vi "Device tester (juicer).vi"() -> ()   [LabVIEW 2015]
uses:
  Device/Typedefs/Juicer.ctl
  Rack/Typedefs/OutputRequest refnum.ctl
  Rack/Typedefs/OutputRequest.ctl
  Rack/Typedefs/InputData cluster.ctl
  Rack/Methods/Port drivers/DigitalInput-DataCluster.ctl
  Device/Typedefs/Valve.ctl
  Rack/Methods/Rack-Init.vi
  Device/Methods/Juicer-Init.vi
  Device/Methods/Valve-Init.vi
  Rack/Methods/Rack-Config.vi
  Rack/Methods/Rack-Start.vi
  Device/Methods/Valve-Open.vi
  Device/Methods/Valve-Close.vi
  Device/Methods/Valve-Pulse.vi
  Device/Methods/Juicer-ChangeMode.vi
  Rack/Methods/Rack-Stop.vi
panel:
  in  "Valve #":i32=1
  out "Valve refs":refnum<vi>[](array[refnum])
  in  "Valve 12":T1={"Settings"={"Timestamp port name"="dsub_panel.p9.7", "Port name"="juicer.valve12", "Port index"=-1}, "OutputRequest event ref"=refnum, "InputData reference"=refnum, "Default length (ms)"=100}
  in  "Valve 11":T1={"Settings"={"Timestamp port name"="dsub_panel.p9.7", "Port name"="juicer.valve11", "Port index"=-1}, "OutputRequest event ref"=refnum, "InputData reference"=refnum, "Default length (ms)"=100}
  in  "Valve 10":T1={"Settings"={"Timestamp port name"="dsub_panel.p9.7", "Port name"="juicer.valve10", "Port index"=-1}, "OutputRequest event ref"=refnum, "InputData reference"=refnum, "Default length (ms)"=100}
  in  "Valve 9":T1={"Settings"={"Timestamp port name"="dsub_panel.p9.7", "Port name"="juicer.valve9", "Port index"=-1}, "OutputRequest event ref"=refnum, "InputData reference"=refnum, "Default length (ms)"=100}
  in  "Valve 8":T1={"Settings"={"Timestamp port name"="dsub_panel.p9.7", "Port name"="juicer.valve8", "Port index"=-1}, "OutputRequest event ref"=refnum, "InputData reference"=refnum, "Default length (ms)"=100}
  in  "Valve 7":T1={"Settings"={"Timestamp port name"="dsub_panel.p9.7", "Port name"="juicer.valve7", "Port index"=-1}, "OutputRequest event ref"=refnum, "InputData reference"=refnum, "Default length (ms)"=100}
  in  "Valve 6":T1={"Settings"={"Timestamp port name"="dsub_panel.p9.7", "Port name"="juicer.valve6", "Port index"=-1}, "OutputRequest event ref"=refnum, "InputData reference"=refnum, "Default length (ms)"=100}
  in  "Valve 5":T1={"Settings"={"Timestamp port name"="dsub_panel.p9.7", "Port name"="juicer.valve5", "Port index"=-1}, "OutputRequest event ref"=refnum, "InputData reference"=refnum, "Default length (ms)"=100}
  in  "Valve 4":T1={"Settings"={"Timestamp port name"="dsub_panel.p9.7", "Port name"="juicer.valve4", "Port index"=-1}, "OutputRequest event ref"=refnum, "InputData reference"=refnum, "Default length (ms)"=100}
  in  "Valve 3":T1={"Settings"={"Timestamp port name"="dsub_panel.p9.7", "Port name"="juicer.valve3", "Port index"=-1}, "OutputRequest event ref"=refnum, "InputData reference"=refnum, "Default length (ms)"=100}
  in  "Valve 2":T1={"Settings"={"Timestamp port name"="dsub_panel.p9.7", "Port name"="juicer.valve2", "Port index"=-1}, "OutputRequest event ref"=refnum, "InputData reference"=refnum, "Default length (ms)"=100}
  in  "Valve 1":T1={"Settings"={"Timestamp port name"="BNC_panel.P0.0", "Port name"="BNC_panel.P0.1", "Port index"=-1}, "OutputRequest event ref"=refnum, "InputData reference"=refnum, "Default length (ms)"=100}
  in  "Juicer":T3={"Mode"=enum."Off", "Settings"={"Bleed #1 port index"=-1, "Bleed #1 port name"="juicer.bleed1", "Bleed #2 port name"="juicer.bleed2", "Bleed #2 port index"=-1, "Flush port name"="juicer.flush", "Flush port index"=-1, "Purge port name"="juicer.purge", "Purge port index"=-1, "Timestamp port name"="dsub_panel.p9.7"}, "OutputRequest event ref"=refnum, "InputData reference"=refnum}
  in  "# repeats":u32=200
  in  "Serial pulse":bool
  in  "Juicer mode":enum16{"off", "reward", "flush", "purge"}(ring)
  in  "Duration (0 for default)":i32
  in  "stop":bool
  in  "Close all":bool
  in  "Close":bool
  in  "Open":bool
  in  "Pulse":bool
  # "Remember to stop this VI before starting\nother behavior VIs that use the juicer!"
  # "(must be on same NI card)"
  # "(must be on same NI card)"
  # "(must be on same NI card)"
  # "(must be on same NI card)"
  # "(must be on same NI card)"
  # "(must be on same NI card)"
  # "(must be on same NI card)"
  # "(must be on same NI card)"
  # "(must be on same NI card)"
  # "(must be on same NI card)"
  # "(must be on same NI card)"
  # "(must be on same NI card)"
  # "(must be on same NI card)"
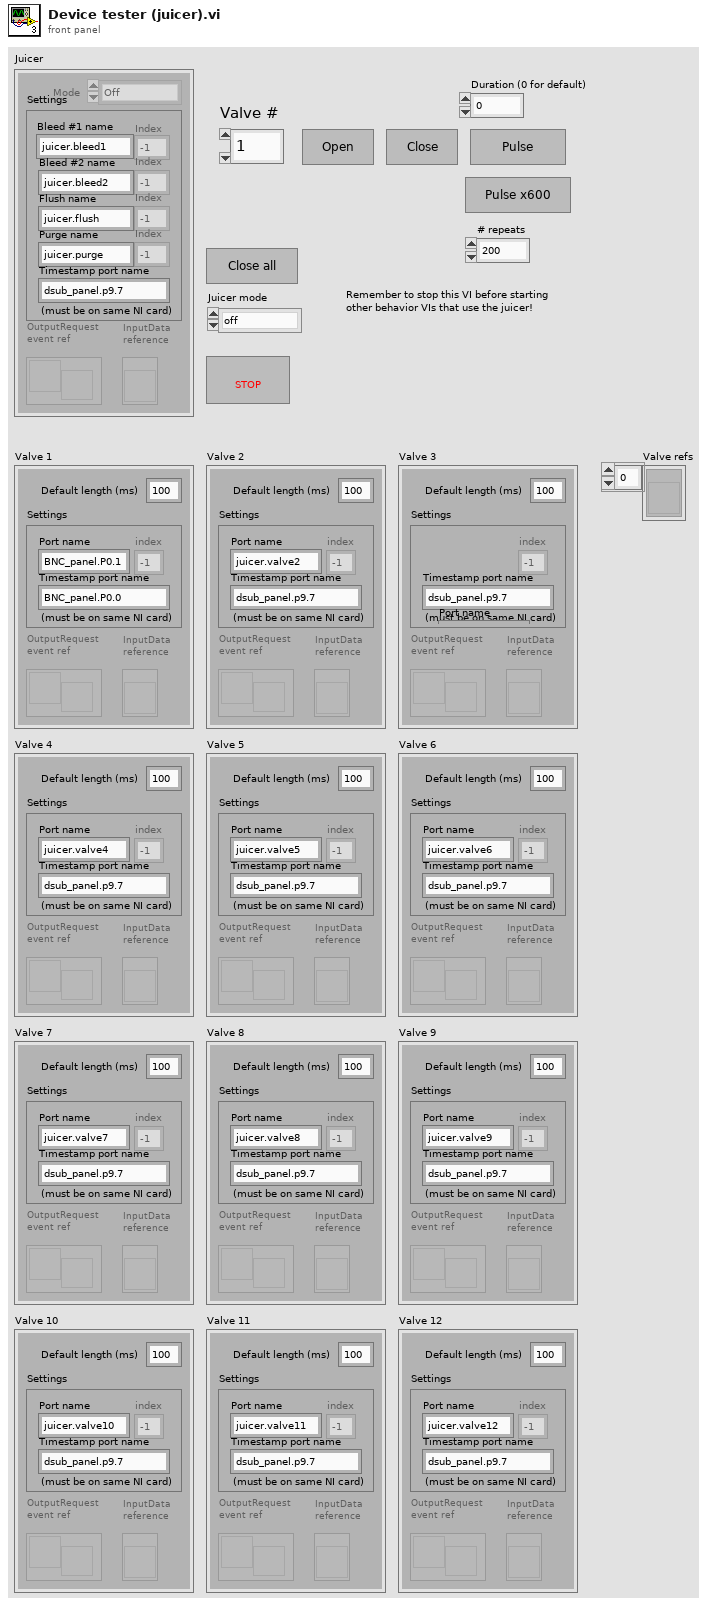
[diagram p1: front panel]
types:
  T1 = typedef "Valve.ctl" = cluster{"Settings":cluster{"Timestamp port name":string, "Port name":string, "Port index":i32}, "OutputRequest event ref":T2, "InputData reference":refnum<vi>, "Default length (ms)":i32}
  T2 = typedef "OutputRequest refnum.ctl" = refnum<user-event>
  T3 = typedef "Juicer.ctl" = cluster{"Mode":enum16{"Off", "Juice/reward", "Water flush", "Air purge"}, "Settings":cluster{"Bleed #1 port index":i32, "Bleed #1 port name":string, "Bleed #2 port name":string, "Bleed #2 port index":i32, "Flush port name":string, "Flush port index":i32, "Purge port name":string, "Purge port index":i32, "Timestamp port name":string}, "OutputRequest event ref":T2, "InputData reference":refnum<vi>}
  T4 = typedef "Rack driver configuration cluster.ctl" = cluster{"DigitalInput":T5, "DigitalOutput":T6, "FileOutput":T7, "AnalogOutput":T8, "DataSocketOutput":T9}
  T5 = typedef "DigitalInput-Configuration.ctl" = cluster{"Lines":tag[], "Refresh period (ms)":u32}
  T6 = typedef "DigitalOutput-Configuration.ctl" = cluster{"Output Lines":tag[], "DO timestamp lines":tag[], "Timestamp lines":tag[]}
  T7 = typedef "FileOutput-Configuration.ctl" = cluster{"Logfile path":path}
  T8 = typedef "AnalogOutput-Configuration.ctl" = cluster{"Output Lines":tag[], "AO timestamp lines":tag[]}
  T9 = typedef "DataSocketOutput-Configuration.ctl" = cluster{"DataSocket URL":string}
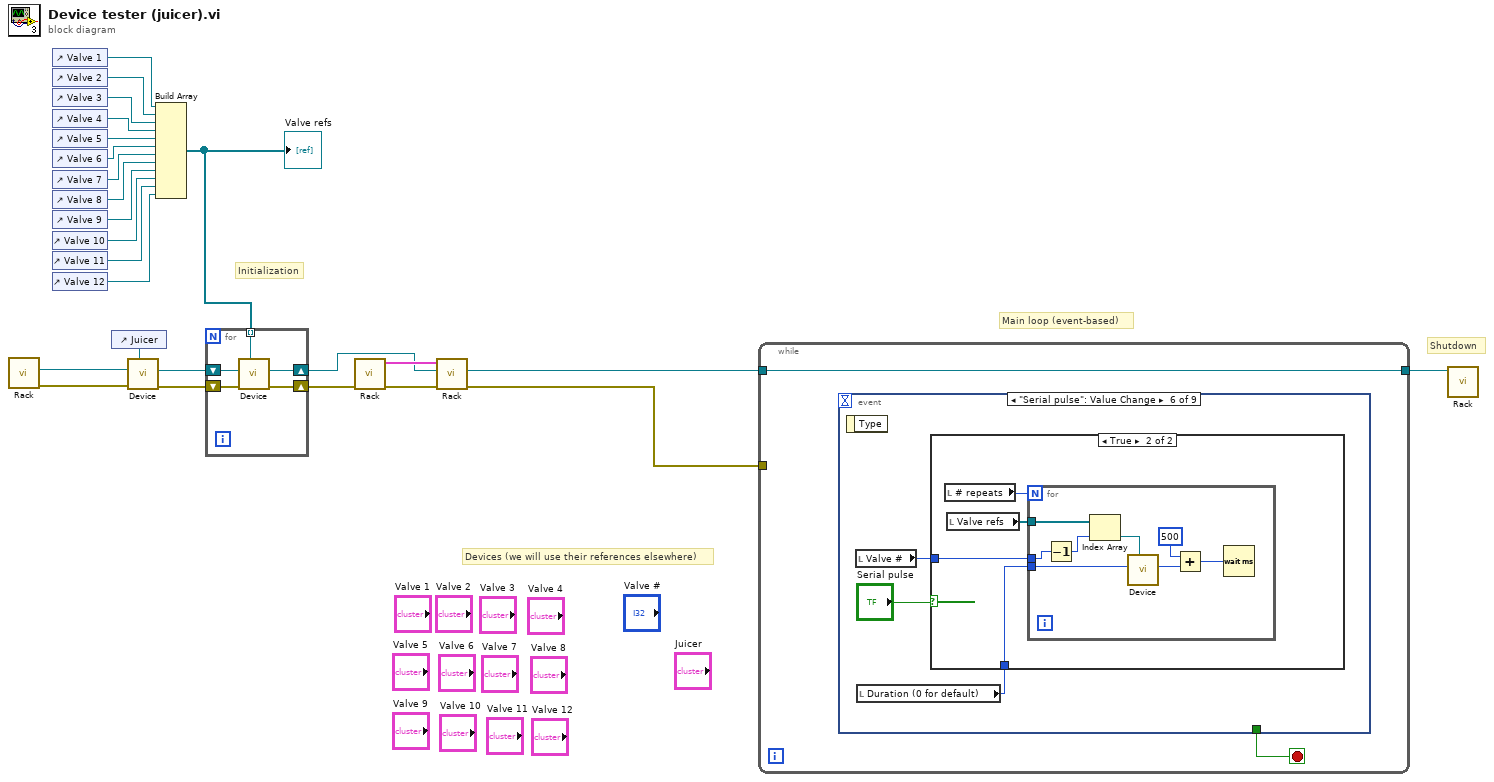
[diagram p0: block diagram]
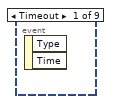
[diagram p2: hidden frame]
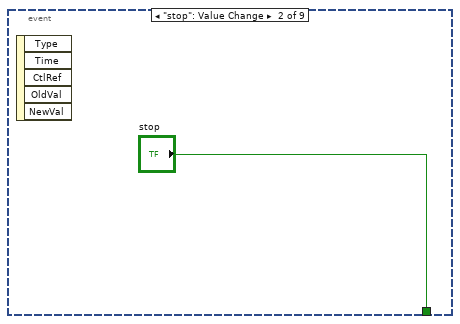
[diagram p3: hidden frame]
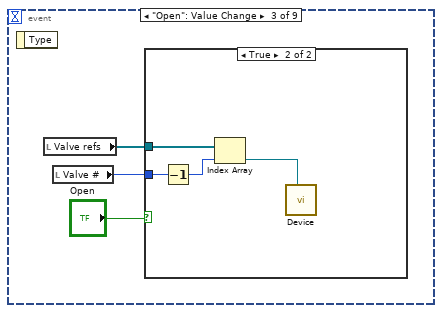
[diagram p4: hidden frame]
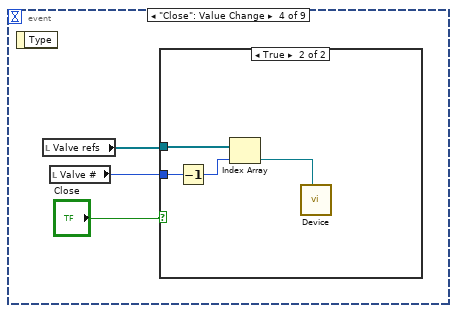
[diagram p6: hidden frame]
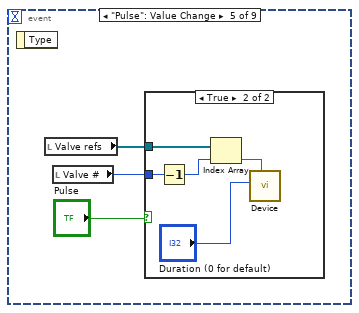
[diagram p8: hidden frame]
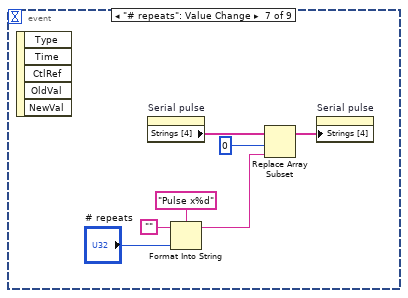
[diagram p11: hidden frame]
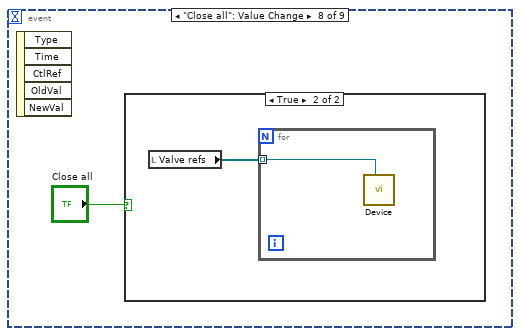
[diagram p12: hidden frame]
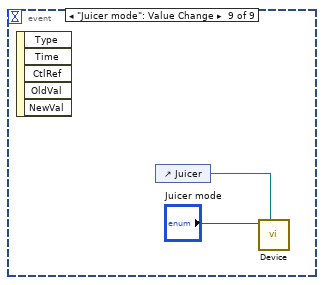
[diagram p14: hidden frame]
diagram:
  # "Main loop (event-based)"
  # "Shutdown"
  # "Initialization"
  # "Devices (we will use their references elsewhere)"
  n1 = call-poly "Rack.vi"() -> ("error out"=w25:errorcluster, "OutputRequest\nevent ref"=w21:T2)  [unwired: 10 in]
  n2 = control-ref of="Valve 1"() -> (w18:refnum<vi>)
  n3 = control-ref of="Valve 2"() -> (w17:refnum<vi>)
  n4 = control-ref of="Valve 3"() -> (w16:refnum<vi>)
  n5 = control-ref of="Valve 4"() -> (w15:refnum<vi>)
  n6 = control-ref of="Valve 5"() -> (w14:refnum<vi>)
  n7 = control-ref of="Valve 6"() -> (w7:refnum<vi>)
  n8 = control-ref of="Valve 7"() -> (w8:refnum<vi>)
  n9 = control-ref of="Valve 8"() -> (w9:refnum<vi>)
  n10 = control-ref of="Valve 9"() -> (w10:refnum<vi>)
  n11 = control-ref of="Valve 10"() -> (w11:refnum<vi>)
  n12 = control-ref of="Valve 11"() -> (w12:refnum<vi>)
  n13 = control-ref of="Valve 12"() -> (w13:refnum<vi>)
  n14 = control-ref of="Juicer"() -> (w19:refnum<vi>)
  n15 = call-poly "Device.vi"("Device reference"=w19, "error in (no error)"=w25, "OutputRequest event ref"=w21) -> ("error out"=w6:errorcluster, "OutputRequest (dup)"=w4:T2)  [unwired: 6 in, 1 out]
  n16 = Build Array(w18, w17, w16, w15, w14, w7, w8, w9, w10, w11, w12, w13) -> (w1:refnum<vi>[])
  "Valve refs" <- w1
  n17 = for {
    shift-right: [w27] -> w5
    shift-left: w6 -> [w30]
    shift-right: [w28] -> w3
    shift-left: w4 -> [w29]
    tunnel: w1 -> [w26] mode=indexing
    n18 = call-poly "Device.vi"("Device reference"=w26, "error in (no error)"=w30, "OutputRequest event ref"=w29) -> ("error out"=w27:errorcluster, "OutputRequest (dup)"=w28:T2)  [unwired: 6 in, 1 out]
  }
  n19 = call-poly "Rack.vi"("error in (no error)"=w5) -> ("error out"=w24:errorcluster, "Configuration"=w23:T4)  [unwired: 9 in]
  n20 = call-poly "Rack.vi"("error in (no error)"=w24, "OutputRequest event ref"=w3, "Configuration"=w23) -> ("error out"=w2:errorcluster, "OutputRequest event ref (dup)"=w20:T2)  [unwired: 7 in]
  n21 = while {
    tunnel: w20 -> [w31]
    tunnel: [w31] -> w22
    tunnel: w2 -> [_]
    stop <- w32 stop-if-true
    n22 = event shown="[5] \"Serial pulse\": Value Change" {
      selector: _ -> [_ _ _ _ _ _ _ _ _]
      dyn-events: _ -> [_ _ _ _ _ _ _ _ _]
      timeout: _ -> [_ _ _ _ _ _ _ _ _]
      tunnel: [_ "stop" _ _ _ _ _ _ _] -> w32
      event Timeout {
        n23 = event-data() -> ()  [unwired: 1 in, 2 out]
      }
      event "stop": Value Change {
        n24 = event-data() -> ()  [unwired: 1 in, 5 out]
      }
      event "Open": Value Change {
        n25 = event-data() -> ()  [unwired: 1 in, 1 out]
        n26 = local read "Valve refs"() -> (w34:refnum<vi>[])
        n27 = local read "Valve #"() -> (w35:i32)
        n28 = case shown="True" "Open" {
          tunnel: w35 -> [_ w39]
          tunnel: w34 -> [_ w40]
          frame False {
          }
          frame True {
            n29 = Decrement(x=w39) -> (x-1=w38:i32)
            n30 = Index Array(array=w40, index=w38) -> (element=w37:refnum<vi>)
            n31 = call-poly "Device.vi"("Device reference"=w37) -> ()  [unwired: 10 in, 1 out]
          }
        }
      }
      event "Close": Value Change {
        n32 = event-data() -> ()  [unwired: 1 in, 1 out]
        n33 = local read "Valve refs"() -> (w41:refnum<vi>[])
        n34 = local read "Valve #"() -> (w42:i32)
        n35 = case shown="True" "Close" {
          tunnel: w42 -> [_ w46]
          tunnel: w41 -> [_ w47]
          frame False {
          }
          frame True {
            n36 = Decrement(x=w46) -> (x-1=w45:i32)
            n37 = Index Array(array=w47, index=w45) -> (element=w44:refnum<vi>)
            n38 = call-poly "Device.vi"("Device reference"=w44) -> ()  [unwired: 10 in, 1 out]
          }
        }
      }
      event "Pulse": Value Change {
        n39 = event-data() -> ()  [unwired: 1 in, 1 out]
        n40 = local read "Valve refs"() -> (w48:refnum<vi>[])
        n41 = local read "Valve #"() -> (w50:i32)
        n42 = case shown="True" "Pulse" {
          tunnel: w50 -> [_ w53]
          tunnel: w48 -> [_ w51]
          frame False {
          }
          frame True {
            n43 = Decrement(x=w53) -> (x-1=w54:i32)
            n44 = Index Array(array=w51, index=w54) -> (element=w52:refnum<vi>)
            n45 = call-poly "Device.vi"("Device reference"=w52, "Duration"="Duration (0 for default)") -> ()  [unwired: 8 in, 2 out]
          }
        }
      }
      event "Serial pulse": Value Change {
        n46 = event-data() -> ()  [unwired: 1 in, 1 out]
        n47 = local read "Valve #"() -> (w58:i32)
        n48 = local read "Duration (0 for default)"() -> (w56:i32)
        n49 = case shown="True" "Serial pulse" {
          tunnel: w58 -> [_ w62]
          tunnel: w56 -> [_ w61]
          frame False {
          }
          frame True {
            n50 = local read "# repeats"() -> (w60:u32)
            n51 = local read "Valve refs"() -> (w59:refnum<vi>[])
            n52 = for {
              N: w60 -> [_]
              tunnel: w62 -> [w65]
              tunnel: w61 -> [w70]
              tunnel: w59 -> [w64]
              n53 = Decrement(x=w65) -> (x-1=w66:i32)
              n54 = Index Array(array=w64, index=w66) -> (element=w63:refnum<vi>)
              n55 = call-poly "Device.vi"("Device reference"=w63, "Duration"=w70) -> ("Actual duration"=w69:i32)  [unwired: 8 in, 1 out]
              n56 = Add(x=500, y=w69) -> (x+y=w67:i32)
              n57 = Wait (ms)(milliseconds to wait=w67) -> ()  [unwired: 1 out]
            }
          }
        }
      }
      event "# repeats": Value Change {
        n58 = event-data() -> ()  [unwired: 1 in, 5 out]
        n59 = property on="Serial pulse" class="Bool"() -> ("Strings [4]"=w77:string[])  [unwired: 2 in, 2 out]
        n60 = Format Into String(format string="Pulse x%d", initial string="", "# repeats") -> (resulting string=w71:string)  [unwired: 1 in, 1 out]
        n61 = Replace Array Subset(array=w77, new element=w71, index=0) -> (w76:string[])
        n62 = property on="Serial pulse" class="Bool"("Strings [4]"=w76) -> ()  [unwired: 2 in, 2 out]
      }
      event "Close all": Value Change {
        n63 = event-data() -> ()  [unwired: 1 in, 5 out]
        n64 = case shown="True" "Close all" {
          frame False {
          }
          frame True {
            n65 = local read "Valve refs"() -> (w79:refnum<vi>[])
            n66 = for {
              tunnel: w79 -> [w80] mode=indexing
              n67 = call-poly "Device.vi"("Device reference"=w80) -> ()  [unwired: 10 in, 1 out]
            }
          }
        }
      }
      event "Juicer mode": Value Change {
        n68 = event-data() -> ()  [unwired: 1 in, 5 out]
        n69 = control-ref of="Juicer"() -> (w81:refnum<vi>)
        n70 = call-poly "Device.vi"("Device reference"=w81, "Mode"="Juicer mode") -> ()  [unwired: 9 in, 1 out]
      }
    }
  }
  n71 = call-poly "Rack.vi"("OutputRequest channel"=w22) -> ()  [unwired: 10 in, 1 out]
